vi "VISA Write with Terminator.vi"(2 "error in (no error)":errorcluster, 3 "String to Write":string, 4 "VISA session":refnum<visa-resource-name>) -> (0 "error out":errorcluster, 1 "dup VISA session":refnum<visa-resource-name>)   [LabVIEW 2019]
doc: "Does a GPIB write and appends the terminator if necessay. This should be super seded with message based VISA settings in later versions of VISA.\nScott Hannahs, <sth@magnet.fsu.edu> NHMFL-FSU, May 2003"
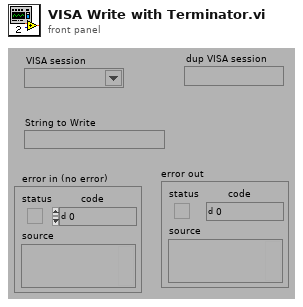
[diagram p1: front panel]
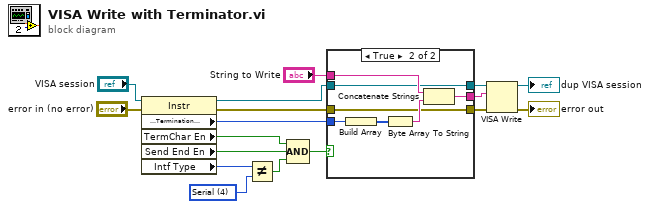
[diagram p0: block diagram]
diagram:
  w1 = u16 4 items=["GPIB"=1, "VXI"=2, "GPIB-VXI"=3, "Serial"=4, "PXI"=5, "TCPIP"=6, "USB"=7, "FireWire"=9] ("Interface Information:Interface Type")
  n1 = property class="Instr"(reference="VISA session", error in="error in (no error)") -> (reference out=w10:refnum<visa-resource-name>, error out=w7:errorcluster, "Message Based Settings:Termination Character"=w12:u8, "TermChar En"=w6:bool, "Send End En"=w5:bool, "Intf Type"=w4:u16)
  n2 = Not Equal?(x=w4, y=w1) -> (x != y?=w3:bool)
  n3 = Compound Arithmetic op=AND(w6, w5, w3) -> (w2:bool)
  n4 = case shown="True" w2 {
    tunnel: "String to Write" -> [w20 w24]
    tunnel: w12 -> [_ w26]
    tunnel: [w20 w23] -> w11
    tunnel: [w19 w22] -> w9
    tunnel: w10 -> [w19 w22]
    tunnel: [w18 w21] -> w8
    tunnel: w7 -> [w18 w21]
    frame False {
    }
    frame True {
      n5 = Build Array(w26) -> (w27:u8[])
      n6 = Byte Array To String(unsigned byte array=w27) -> (string=w25:string)
      n7 = Concatenate Strings(w24, w25) -> (w23:string)
    }
  }
  n8 = VISA Write(VISA resource name=w9, write buffer=w11, error in (no error)=w8) -> (VISA resource name out=→"dup VISA session":refnum<visa-resource-name>, error out=→"error out":errorcluster)  [unwired: 1 out]
